vi "Auth.vi"(7 "Values In":refnum<class "Values.lvclass">, 8 "error in (no error)":errorcluster, 9 "Anonymous (F)":bool, 10 "User (None)":refnum<class "User.lvclass">, 11 "Security in":refnum<class "Security.lvclass">) -> (0 "error out":errorcluster, 3 "Security out":refnum<class "Security.lvclass">, 5 "Values":refnum<class "Values.lvclass">)   [LabVIEW 2020, in "HTTP Server.lvlib" / "Security.lvclass"]
uses:
  Security.lvclass
  User/User.lvclass
  Values/Values.lvclass
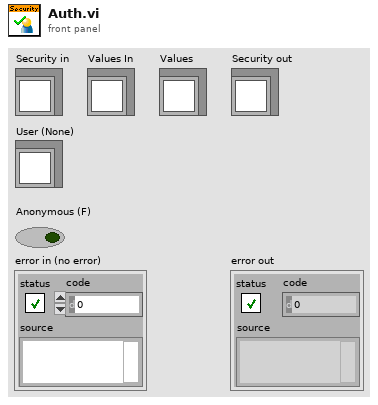
[diagram p1: front panel]
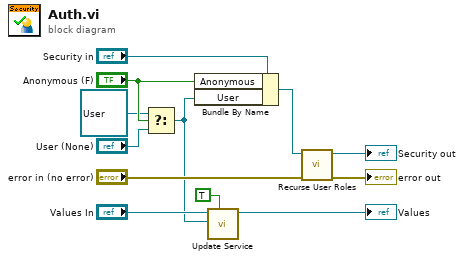
[diagram p0: block diagram]
diagram:
  n1 = Select(t=refnum<class "User.lvclass"> refnum, s="Anonymous (F)", f="User (None)") -> (s? t:f=w1:refnum<class "User.lvclass">)
  n2 = Bundle By Name(cluster="Security in", "Anonymous"="Anonymous (F)", "User"=w1) -> (w11:refnum<class "Security.lvclass">)
  n3 = call "Update Service.vi"("Overwrite? (F)"=TRUE, "Service"=w1, "Values in"="Values In") -> ("Values out"=→"Values":refnum<class "Values.lvclass">)  [unwired: 7 in, 1 out]
  n4 = call "Recurse User Roles.vi"("error in (no error)"="error in (no error)", "Security in"=w11) -> ("error out"=→"error out":errorcluster, "Security out"=→"Security out":refnum<class "Security.lvclass">)  [unwired: 8 in]
